vi "PC_AIChar_v3.vi"() -> ()   [LabVIEW 2020]
uses:
  TypeDefs/UIStateDefEnum.ctl
  <vilib>/measure/maspectr.llb/Power Spectrum and PSD Export Mode.ctl
  <vilib>/NI/STM/TCP/Read Meta Data (TCP Clst).vi
  <vilib>/NI/STM/TCP/Read Message (TCP).vi
  <vilib>/NI/STM/TCP/Read Meta Data (TCP Ref).vi
  <vilib>/measure/maspectr.llb/FFT Power Spectrum and PSD for 1 Chan.vi
  <vilib>/Analysis/5stat.llb/RMS (DBL).vi
  <vilib>/Analysis/baseanly.llb/Mean (DBL).vi
  <vilib>/NI/STM/TCP/Get Connection Reference (TCP).vi
  <vilib>/NI/STM/NI STM.lvlib
  <vilib>/Analysis/NI_AALBase.lvlib
  <vilib>/measure/NI_MAPro.lvlib
  <vilib>/Analysis/NI_AALPro.lvlib
  Components/Spectra/Spectra.lvlib
  <vilib>/Analysis/1siggen.llb/Ramp Pattern by Delta.vi
  <vilib>/Utility/file.llb/Write Delimited Spreadsheet (DBL).vi
panel:
  in  "SaveData":bool
  in  "Select\nTarget":enum16{"myRIO", "cRIO"}(ring)
  out "Analysis Loop \ntime [s]":dbl format="%#.4g"
  out "Analysis \ntime-span [s]":dbl format="%.2f"
  out "# of elements \nremoved":i32
  in  "Pause Charts":bool
  in  "Clear charts":bool
  out "RT target \nloop \ntime [s]":dbl=0.0002
  out "Data length \n[count]":i32
  out "Mean [V]":dbl format="%#.6f"
  out "RMS / \nStd. Dev. [mV]":dbl format="%#.6f"
  out "Spectra plots":cluster{"f0":dbl, "df":dbl, "magnitude":dbl[]}[](graph)
  out "Histogram Graph":T1(graph)
  out "STM Loop \ntime [s]":dbl format="%#.4g"
  in  "System Stop Button":bool
  out "Data":dbl[][](graph)
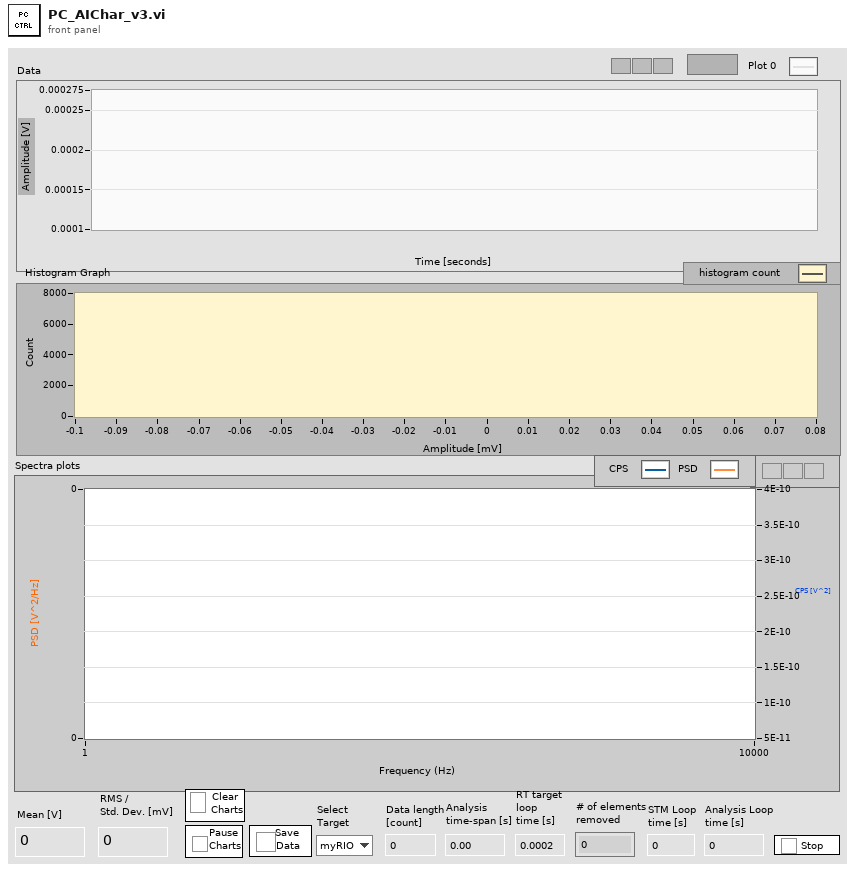
[diagram p1: front panel]
types:
  T1 = cluster{"X Values":dbl[], "Histogram: h(x)":i32[]}
  T2 = typedef "UIStateDefEnum.ctl" = enum16{"Wait", "Initialize", "Clear", "SaveData", "Stop"}
  T3 = typedef "NI STM.lvlib/TCP Connection Info.ctl" = cluster{"connection ID":refnum<k5>, "meta data":T4[]}
  T4 = typedef "NI STM.lvlib/MetaDataElement.ctl" = string
  T5 = typedef "NI_MAPro.lvlib/Power Spectrum and PSD Export Mode.ctl" = u16
  T6 = typedef "imagedata.ctl" = cluster{"image type":i32, "image depth":i32, "image":u8[], "mask":u8[], "colors":u32[], "Rectangle":cluster{"left":i16, "top":i16, "right":i16, "bottom":i16}}
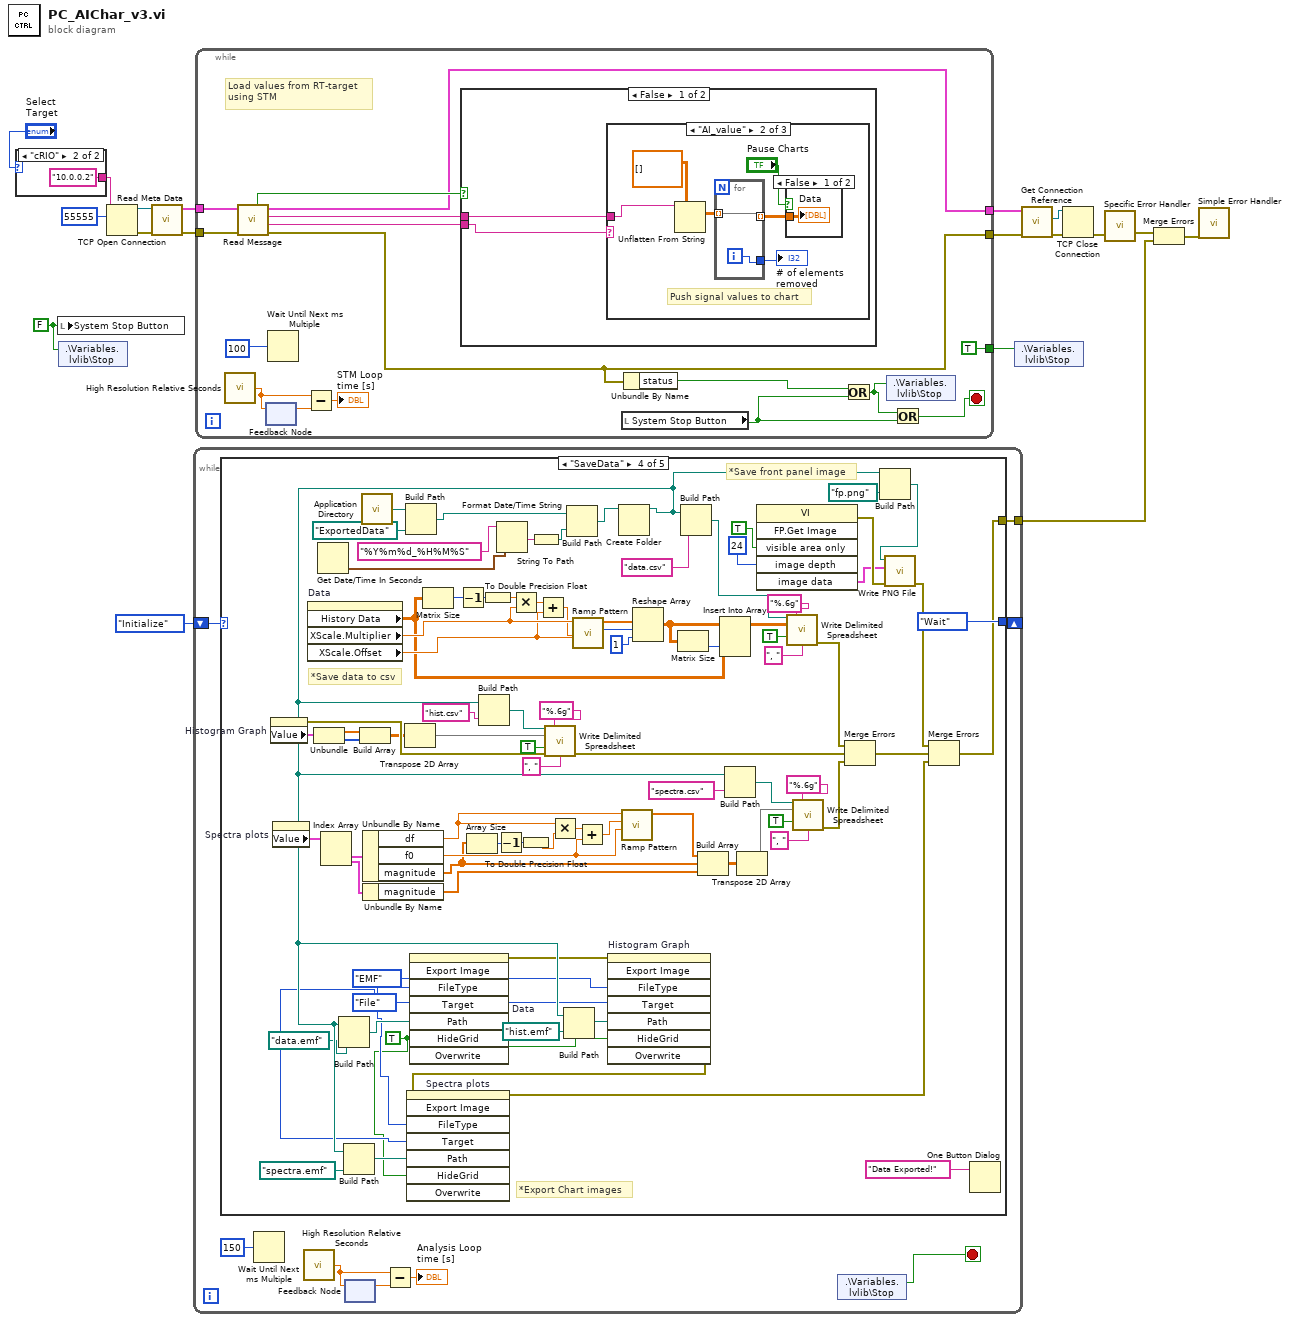
[diagram p0: block diagram]
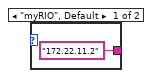
[diagram p2: hidden frame]
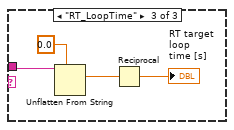
[diagram p5: hidden frame]
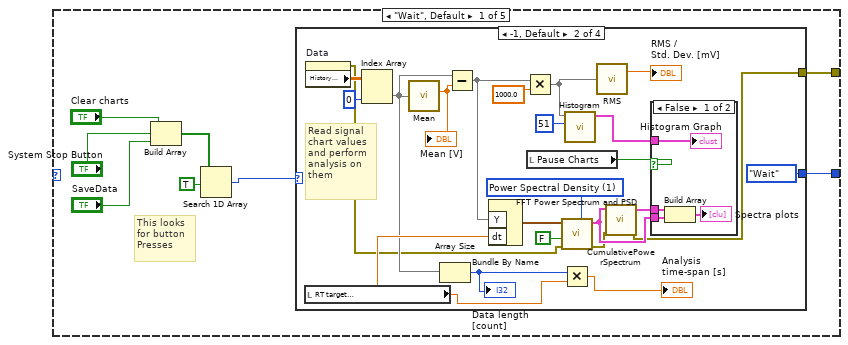
[diagram p7: hidden frame]
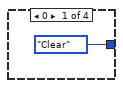
[diagram p8: hidden frame]
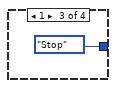
[diagram p10: hidden frame]
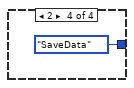
[diagram p11: hidden frame]
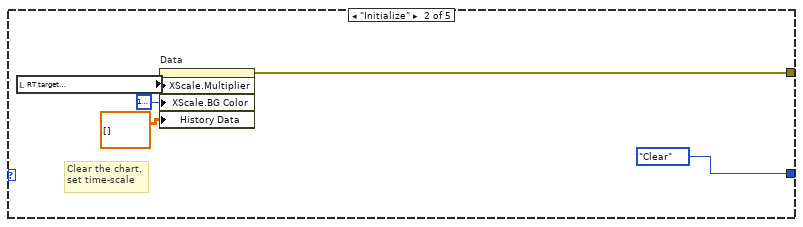
[diagram p12: hidden frame]
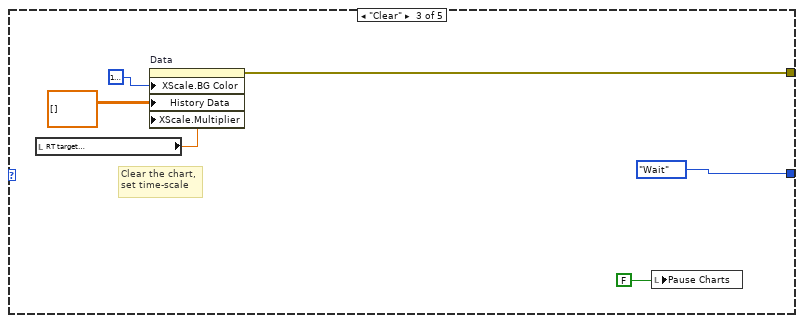
[diagram p13: hidden frame]
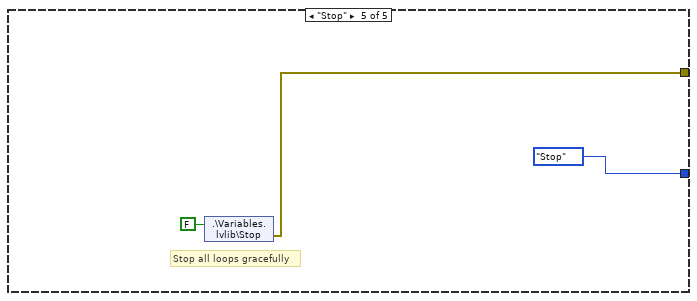
[diagram p14: hidden frame]
diagram:
  w7 = FALSE ("System Stop Button")
  n1 = case shown="\"cRIO\"" "Select\nTarget" {
    tunnel: ["172.22.11.2" ("address") "10.0.0.2" ("address")] -> w17
    frame "myRIO", Default {
    }
    frame "cRIO" {
    }
  }
  n2 = local write "System Stop Button"(w7) -> ()
  n3 = shared-variable ".\\Variables.lvlib\\Stop"(w7) -> ()  [unwired: 1 in, 1 out]
  n4 = TCP Open Connection(address=w17, remote port or service name=u16 55555) -> (connection ID=w16:refnum<k5>, error out=w15:errorcluster)  [unwired: 3 in]
  n5 = call-poly <vilib>:"Read Meta Data.vi"("error in"=w15, "connection ID"=w16) -> ("error out"=w13:errorcluster, "connection info out"=w14:T3)  [unwired: 7 in, 1 out]
  n6 = while {
    shift-right: [w26] -> _
    shift-left: UIStateDefEnum."Initialize" ("UIStateDefEnum") -> [w27]
    tunnel: [w21] -> w1
    stop <- w25 stop-if-true
    n7 = case shown="\"SaveData\"" w27 {
      tunnel: [w31 UIStateDefEnum."Clear" ("UIStateDefEnum") UIStateDefEnum."Wait" ("UIStateDefEnum") UIStateDefEnum."Wait" ("UIStateDefEnum") UIStateDefEnum."Stop" ("UIStateDefEnum")] -> w26
      tunnel: [w29 w67 w72 w78 w163] -> w21
      frame "Wait", Default {
        # "This looks \nfor button \nPresses"
        n8 = Build Array "Build Array"("Clear charts", "System Stop Button", "SaveData") -> (w36:bool[])
        n9 = Search 1D Array(1D array=w36, element=TRUE) -> (index of element=w32:i32)  [unwired: 1 in]
        n10 = case shown="-1, Default" w32 {
          tunnel: [UIStateDefEnum."Clear" ("UIStateDefEnum") UIStateDefEnum."Wait" ("UIStateDefEnum") UIStateDefEnum."Stop" ("UIStateDefEnum") UIStateDefEnum."SaveData" ("UIStateDefEnum")] -> w31
          tunnel: [_ w38 _ _] -> w29
          frame 0 {
          }
          frame -1, Default {
            w56 = T5 1 items=["Power Spectrum", "Power Spectral Density"] ("export mode")
            # "Read signal\nchart values\nand perform\nanalysis on \nthem"
            n11 = local read "RT target \nloop \ntime [s]"() -> (w49:dbl)
            n12 = property on="Data" class="WFChart (strict)"() -> (error out=w39:errorcluster, "History Data"=w54:dbl[][])  [unwired: 2 in, 1 out]
            n13 = Index Array(array=w54, index (col)=0 ("disabled index (col)")) -> (element=w44:dbl[])  [unwired: 1 in]
            n14 = call-poly <vilib>:"Mean.vi"("X"=w44) -> ("mean"=w55:dbl)  [unwired: 1 out]
            "Mean [V]" <- w55
            n15 = Array Size(array=w44) -> (size(s)=w50:i32)
            "Data length \n[count]" <- w50
            n16 = Subtract(x=w44, y=w55) -> (x-y=w43:dbl[])
            n17 = Bundle By Name("Y"=w43, "dt"=w49) -> (w58:waveform(dbl))  [unwired: 1 in]
            n18 = Multiply(x=w43, y=1000.0) -> (x*y=w45:dbl[])
            n19 = local read "Pause Charts"() -> (w48:bool)
            n20 = call-poly <vilib>:"FFT Power Spectrum and PSD.vi"("export mode"=w56, "error in (no error)"=w39, "dB On (F)"=FALSE, "time signal"=w58) -> ("error out"=w40:errorcluster, "Power Spectrum / PSD"=w41:cluster{"f0":dbl, "df":dbl, "magnitude":dbl[]})  [unwired: 4 in, 2 out]
            n21 = Multiply(x=w50, y=w49) -> (x*y=→"Analysis \ntime-span [s]":dbl)
            n22 = call <vilib>:"Histogram.vi"("intervals"=51, "X"=w45) -> ("Histogram Graph"=w59:T1)  [unwired: 6 in, 3 out]
            n23 = call-poly <vilib>:"RMS.vi"("X"=w45) -> ("rms value"=→"RMS / \nStd. Dev. [mV]":dbl)  [unwired: 1 out]
            n24 = call "CumulativePowerSpectrum.vi"("error in (no error)"=w40, "PSD"=w41) -> ("error out"=w38:errorcluster, "CPS"=w42:cluster{"f0":dbl, "df":dbl, "magnitude":dbl[]})  [unwired: 8 in]
            n25 = case shown="False" w48 {
              tunnel: w59 -> [w64 _]
              tunnel: w42 -> [w63 _]
              tunnel: w41 -> [w61 _]
              frame False {
                n26 = Build Array(w63, w61) -> (→"Spectra plots":cluster{"f0":dbl, "df":dbl, "magnitude":dbl[]}[])
                "Histogram Graph" <- w64
              }
              frame True {
              }
            }
          }
          frame 1 {
          }
          frame 2 {
          }
        }
      }
      frame "Initialize" {
        # "Clear the chart,\nset time-scale"
        n27 = local read "RT target \nloop \ntime [s]"() -> (w70:dbl)
        n28 = property on="Data" class="WFChart (strict)"("XScale.Multiplier"=w70, "XScale.BG Color"=u32 16777216 ("X Scale.Marker Colors:BG Color"), "History Data"=dbl[][] []) -> (error out=w67:errorcluster)  [unwired: 2 in, 1 out]
      }
      frame "Clear" {
        # "Clear the chart,\nset time-scale"
        n29 = local read "RT target \nloop \ntime [s]"() -> (w73:dbl)
        n30 = property on="Data" class="WFChart (strict)"("XScale.BG Color"=u32 16777216 ("X Scale.Marker Colors:BG Color"), "History Data"=dbl[][] [], "XScale.Multiplier"=w73) -> (error out=w72:errorcluster)  [unwired: 2 in, 1 out]
        n31 = local write "Pause Charts"(FALSE ("Pause Charts")) -> ()
      }
      frame "SaveData" {
        w94 = TRUE ("Hide Grid")
        w95 = enum32{"File", "Clipboard"}."File" ("Target")
        w96 = enum32{"BMP", "EPS", "EMF", "PICT"}."EMF" ("File Type")
        # "*Export Chart images"
        # "*Save front panel image"
        # "*Save data to csv"
        n32 = property on="Histogram Graph" class="XYGraph (strict)"() -> (error out=w154:errorcluster, "Value"=w132:T1)  [unwired: 2 in, 1 out]
        n33 = property on="Spectra plots" class="WFGraph (strict)"() -> ("Value"=w136:cluster{"f0":dbl, "df":dbl, "magnitude":dbl[]}[])  [unwired: 2 in, 2 out]
        n34 = property on="Data" class="WFChart (strict)"() -> ("History Data"=w105:dbl[][], "XScale.Multiplier"=w115:dbl, "XScale.Offset"=w110:dbl)  [unwired: 2 in, 2 out]
        n35 = Unbundle(w132) -> ("X Values"=w133:dbl[], "Histogram: h(x)"=w134:i32[])
        n36 = Get Date/Time In Seconds() -> (seconds since 1Jan1904=w117:timestamp)
        n37 = Index Array(array=w136) -> (element #1=w137:cluster{"f0":dbl, "df":dbl, "magnitude":dbl[]}, element #2=w138:cluster{"f0":dbl, "df":dbl, "magnitude":dbl[]})  [unwired: 2 in]
        n38 = Build Array(w133, w134) -> (w135:dbl[][])
        n39 = call <vilib>:"Application Directory.vi"() -> ("Application Directory"=w116:path)
        n40 = Unbundle By Name(w137) -> ("df"=w144:dbl, "f0"=w146:dbl, "magnitude"=w141:dbl[])
        n41 = Unbundle By Name(w138) -> ("magnitude"=w139:dbl[])
        n42 = Transpose 2D Array(2D array=w135) -> (transposed array=w153:dbl[][])
        n43 = Build Path(base path=w116, name or relative path=path "ExportedData") -> (appended path=w119:path)
        n44 = Matrix Size(0:w105) -> (1:w106:i32)  [unwired: 1 out]
        n45 = Decrement(x=w106) -> (x-1=w107:i32)
        n46 = Array Size(array=w141) -> (size(s)=w149:i32)
        n47 = To Double Precision Float(number=w107) -> (double precision float=w108:dbl)
        n48 = Decrement(x=w149) -> (x-1=w142:i32)
        n49 = Format Date/Time String(time format string (%c)="%Y%m%d_%H%M%S", seconds (now)=w117) -> (date/time string=w121:string)  [unwired: 1 in]
        n50 = Multiply(x=w108, y=w115) -> (x*y=w109:dbl)
        n51 = To Double Precision Float(number=w142) -> (double precision float=w143:dbl)
        n52 = String To Path(string=w121) -> (path=w120:path)
        n53 = Add(x=w109, y=w110) -> (x+y=w111:dbl)
        n54 = Multiply(x=w144, y=w143) -> (x*y=w145:dbl)
        n55 = Build Path(base path=w119, name or relative path=w120) -> (appended path=w123:path)
        n56 = call-poly <vilib>:"Ramp Pattern.vi"("start"=w110, "end"=w111, "delta"=w115) -> ("samples"=w112:i32, "Ramp Pattern"=w113:dbl[])  [unwired: 6 in, 1 out]
        n57 = Add(x=w145, y=w146) -> (x+y=w147:dbl)
        n58 = Create Folder(path (use dialog)=w123) -> (created path=w159:path)  [unwired: 2 in, 2 out]
        n59 = Build Path(base path=w159, name or relative path=path "data.emf") -> (appended path=w122:path)
        n60 = Build Path(base path=w159, name or relative path=path "spectra.emf") -> (appended path=w125:path)
        n61 = invoke on="Data" class="WFChart (strict)" method="Export Image"("FileType"=w96, "Target"=w95, "Path"=w122, "HideGrid"=w94) -> (error out=w126:errorcluster)  [unwired: 4 in, 7 out]
        n62 = Build Path(base path=w159, name or relative path="hist.csv" ("string")) -> (appended path=w152:path)
        n63 = call-poly <vilib>:"Write Delimited Spreadsheet.vi"("file path (dialog if empty)"=w152, "format (%.3f)"="%.6g", "2D data"=w153, "append to file? (new file:F)"=TRUE, "error in (no error)"=w154, "delimiter (\\t)"=", " ("delimiter (\\t)")) -> ("error out"=w156:errorcluster)  [unwired: 8 in, 1 out]
        n64 = Build Path(base path=w159, name or relative path=path "hist.emf") -> (appended path=w124:path)
        n65 = invoke on="Histogram Graph" class="XYGraph (strict)" method="Export Image"(error in=w126, "FileType"=w96, "Target"=w95, "Path"=w124, "HideGrid"=w94) -> (error out=w127:errorcluster)  [unwired: 3 in, 7 out]
        n66 = invoke on="Spectra plots" class="WFGraph (strict)" method="Export Image"(error in=w127, "FileType"=w96, "Target"=w95, "Path"=w125, "HideGrid"=w94) -> (error out=w140:errorcluster)  [unwired: 3 in, 7 out]
        n67 = call-poly <vilib>:"Ramp Pattern.vi"("start"=w146, "end"=w147, "delta"=w144) -> ("Ramp Pattern"=w148:dbl[])  [unwired: 6 in, 2 out]
        n68 = Reshape Array(w113, w112, 1 ("dimension size")) -> (w114:dbl[][])
        n69 = Matrix Size(0:w114) -> (2:w104:i32)  [unwired: 1 out]
        n70 = Build Path(base path=w159, name or relative path="data.csv" ("string")) -> (appended path=w118:path)
        n71 = Build Array(w148, w141, w139) -> (w150:dbl[][])
        n72 = Insert Into Array(array=w114, index (col)=w104, new element=w105) -> (w151:dbl[][])  [unwired: 1 in]
        n73 = Build Path(base path=w159, name or relative path="spectra.csv" ("string")) -> (appended path=w158:path)
        n74 = Transpose 2D Array(2D array=w150) -> (transposed array=w160:dbl[][])
        n75 = invoke class="VI" method="FP.Get Image"("visible area only"=TRUE ("Visible Area Only"), "image depth"=24 ("Image Depth")) -> (error out=w130:errorcluster, "image data"=w128:T6)  [unwired: 4 in, 4 out]
        n76 = call-poly <vilib>:"Write Delimited Spreadsheet.vi"("file path (dialog if empty)"=w118, "format (%.3f)"="%.6g", "2D data"=w151, "append to file? (new file:F)"=TRUE, "delimiter (\\t)"=", " ("delimiter (\\t)")) -> ("error out"=w155:errorcluster)  [unwired: 9 in, 1 out]
        n77 = call-poly <vilib>:"Write Delimited Spreadsheet.vi"("file path (dialog if empty)"=w158, "format (%.3f)"="%.6g", "2D data"=w160, "append to file? (new file:F)"=TRUE, "delimiter (\\t)"=", " ("delimiter (\\t)")) -> ("error out"=w161:errorcluster)  [unwired: 9 in, 1 out]
        n78 = Merge Errors(w155, w156, w161) -> (w157:errorcluster)
        n79 = Build Path(base path=w159, name or relative path=path "fp.png") -> (appended path=w129:path)
        n80 = call <vilib>:"Write PNG File.vi"("error in (no error)"=w130, "image data"=w128, "path to PNG file"=w129) -> ("error out"=w131:errorcluster)  [unwired: 7 in, 1 out]
        n81 = Merge Errors(w131, w157, w140) -> (w78:errorcluster)
        n82 = One Button Dialog(message="Data Exported!" ("Status....")) -> ()  [unwired: 1 in, 1 out]
      }
      frame "Stop" {
        # "Stop all loops gracefully"
        n83 = shared-variable ".\\Variables.lvlib\\Stop"(FALSE ("Stop")) -> (error out=w163:errorcluster)  [unwired: 1 in]
      }
    }
    n84 = Wait Until Next ms Multiple(millisecond multiple=u32 150) -> ()  [unwired: 1 out]
    n85 = call <vilib>:"High Resolution Relative Seconds.vi"() -> ("relative seconds"=w23:dbl)
    n86 = feedback #1() -> (w24:dbl)  [unwired: 1 in]
    n87 = feedback-in #1(w23) -> ()
    n88 = Subtract(x=w23, y=w24) -> (x-y=→"Analysis Loop \ntime [s]":dbl)
    n89 = shared-variable ".\\Variables.lvlib\\Stop"() -> (w25:bool)  [unwired: 1 in, 1 out]
  }
  n90 = while {
    tunnel: w14 -> [w181]
    tunnel: w13 -> [w180]
    tunnel: [w178] -> w9
    tunnel: [w177] -> w8
    tunnel: [TRUE ("Stop")] -> w5
    stop <- w171 stop-if-true
    # "Load values from RT-target\nusing STM"
    n91 = call <vilib>:"High Resolution Relative Seconds.vi"() -> ("relative seconds"=w173:dbl)
    n92 = call-poly <vilib>:"Read Message.vi"("error in"=w180, "connection info in"=w181) -> ("error out"=w177:errorcluster, "name"=w176:T4, "data string"=w175:string, "connection info out"=w178:T3, "timed out?"=w179:bool)  [unwired: 4 in, 1 out]
    n93 = feedback-in #2(w173) -> ()
    n94 = feedback #2() -> (w174:dbl)  [unwired: 1 in]
    n95 = Wait Until Next ms Multiple(millisecond multiple=u32 100 ("Period")) -> ()  [unwired: 1 out]
    n96 = Subtract(x=w173, y=w174) -> (x-y=→"STM Loop \ntime [s]":dbl)
    n97 = case shown="False" w179 {
      tunnel: w176 -> [w183 _]
      tunnel: w175 -> [w182 _]
      frame False {
        n98 = case shown="\"AI_value\"" w183 {
          tunnel: w182 -> [_ w188 w193]
          frame Default {
          }
          frame "AI_value" {
            # "Push signal values to chart"
            n99 = Unflatten From String(type=dbl[][] [], binary string=w188) -> (value=w187:dbl[][])  [unwired: 3 in, 2 out]
            n100 = for {
              tunnel: w187 -> [w192] mode=indexing
              tunnel: [w192] -> w186 mode=indexing
              tunnel: [w191] -> w185
              i -> [w191]
            }
            "# of elements \nremoved" <- w185
            n101 = case shown="False" "Pause Charts" {
              tunnel: w186 -> [w190 _]
              frame False {
                "Data" <- w190
              }
              frame True {
              }
            }
          }
          frame "RT_LoopTime" {
            n102 = Unflatten From String(type=0.0, binary string=w193) -> (value=w195:dbl)  [unwired: 3 in, 2 out]
            n103 = Reciprocal(x=w195) -> (1/x=→"RT target \nloop \ntime [s]":dbl)
          }
        }
      }
      frame True {
      }
    }
    n104 = local read "System Stop Button"() -> (w170:bool)
    n105 = Unbundle By Name(w177) -> ("status"=w169:bool)
    n106 = Or(x=w169, y=w170) -> (x .or. y?=w168:bool)
    n107 = shared-variable ".\\Variables.lvlib\\Stop"(w168) -> ()  [unwired: 1 in, 1 out]
    n108 = Or(x=w168, y=w170) -> (x .or. y?=w171:bool)
  }
  n109 = shared-variable ".\\Variables.lvlib\\Stop"(w5) -> ()  [unwired: 1 in, 1 out]
  n110 = call-poly <vilib>:"Get Connection Reference.vi"("error in"=w8, "connection info in"=w9) -> ("error out"=w12:errorcluster, "connection ID out"=w11:refnum<k5>)  [unwired: 7 in, 1 out]
  n111 = TCP Close Connection(connection ID=w11, error in (no error)=w12) -> (error out=w10:errorcluster)  [unwired: 1 in, 1 out]
  n112 = call "Specific Error Handler"("Error to Check"=w10) -> ("error out"=w3:errorcluster)  [unwired: 11 in, 3 out]
  n113 = Merge Errors(w3, w1) -> (w2:errorcluster)
  n114 = call <vilib>:"Simple Error Handler.vi"("error in (no error)"=w2) -> ()  [unwired: 4 in, 5 out]
